vi "Lab 9 Exercise 3 - Convert C to F.vi"(11 "deg C":dbl) -> (3 "deg F":dbl)   [LabVIEW 2023]
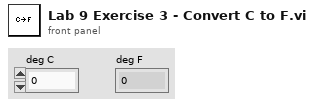
[diagram p1: front panel]
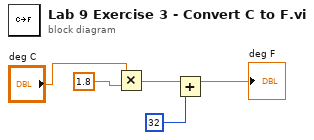
[diagram p0: block diagram]
diagram:
  n1 = Multiply(x="deg C", y=1.8) -> (x*y=w3:dbl)
  n2 = Add(x=w3, y=32) -> (x+y=→"deg F":dbl)
